vi "DriveBase.vi"   [LabVIEW 2015]
uses:
  Robot Global Data.vi
types:
  T1 = cluster{"Reverse":bool, "Speed":dbl, "Left":dbl, "Right":dbl}
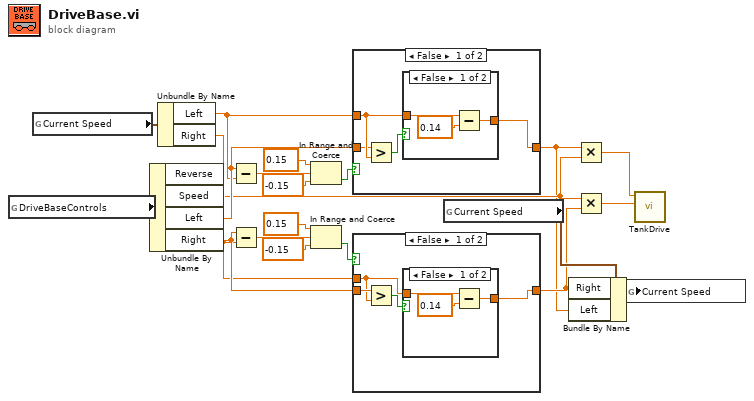
[diagram p0: block diagram]
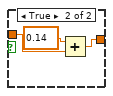
[diagram p2: hidden frame]
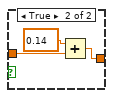
[diagram p4: hidden frame]
diagram:
  n1 = global read "Robot Global Data.vi" "DriveBaseControls"() -> (w21:T1)
  n2 = global read "Robot Global Data.vi" "Current Speed"() -> (w20:cluster{"Left":dbl, "Right":dbl})
  n3 = Unbundle By Name(w21) -> ("Speed"=w2:dbl, "Left"=w12:dbl, "Right"=w9:dbl)  [unwired: 1 out]
  n4 = Unbundle By Name(w20) -> ("Left"=w7:dbl, "Right"=w6:dbl)
  n5 = Subtract(x=w12, y=w7) -> (x-y=w8:dbl)
  n6 = Subtract(x=w9, y=w6) -> (x-y=w13:dbl)
  n7 = In Range and Coerce(upper limit=0.15, x=w8, lower limit=-0.15) -> (In Range?=w19:bool)  [unwired: 1 out]
  n8 = In Range and Coerce(upper limit=0.15, x=w13, lower limit=-0.15) -> (In Range?=w14:bool)  [unwired: 1 out]
  n9 = case shown="False" w19 {
    tunnel: w7 -> [w23 _]
    tunnel: [w25 w32] -> w1
    tunnel: w12 -> [w22 w32]
    frame False {
      n10 = Greater?(x=w22, y=w23) -> (0:w24:bool)
      n11 = case shown="False" w24 {
        tunnel: w23 -> [w27 w31]
        tunnel: [w28 w29] -> w25
        frame False {
          n12 = Subtract(x=w27, y=0.14) -> (x-y=w28:dbl)
        }
        frame True {
          n13 = Add(x=0.14, y=w31) -> (x+y=w29:dbl)
        }
      }
    }
    frame True {
    }
  }
  n14 = case shown="False" w14 {
    tunnel: w6 -> [w34 _]
    tunnel: [w36 w43] -> w3
    tunnel: w9 -> [w35 w43]
    frame False {
      n15 = Greater?(x=w35, y=w34) -> (0:w33:bool)
      n16 = case shown="False" w33 {
        tunnel: w34 -> [w38 w41]
        tunnel: [w37 w40] -> w36
        frame False {
          n17 = Subtract(x=w38, y=0.14) -> (x-y=w37:dbl)
        }
        frame True {
          n18 = Add(x=0.14, y=w41) -> (x+y=w40:dbl)
        }
      }
    }
    frame True {
      # "Tada!"
    }
  }
  n19 = global read "Robot Global Data.vi" "Current Speed"() -> (w5:cluster{"Left":dbl, "Right":dbl})
  n20 = Bundle By Name(cluster=w5, "Right"=w3, "Left"=w1) -> (w4:cluster{"Left":dbl, "Right":dbl})
  n21 = Multiply(x=w1, y=w2) -> (x*y=w11:dbl)
  n22 = Multiply(x=w2, y=w3) -> (x*y=w10:dbl)
  n23 = global write "Robot Global Data.vi" "Current Speed"(w4) -> ()
  n24 = call "TankDrive.vi"("right"=w10, "left"=w11) -> ()  [unwired: 10 in]
